vi "Data_Acquisition.vi"(0 "Upper_Limit":dbl=100.0, 5 "Lower_Bound":dbl, 11 "Error_In":errorcluster) -> (4 "Generated_Number":dbl, 15 "Error_Out":errorcluster)   [LabVIEW 2021]
doc: "This VI Generate data and transmit it to other vi through Queue and stack"
uses:
  Controls/Operation_Select_Queue.ctl
  Controls/Data.ctl
  Controls/Operation_Select_Stack.ctl
  <vilib>/numeric/Random Number (Range) DBL.vi
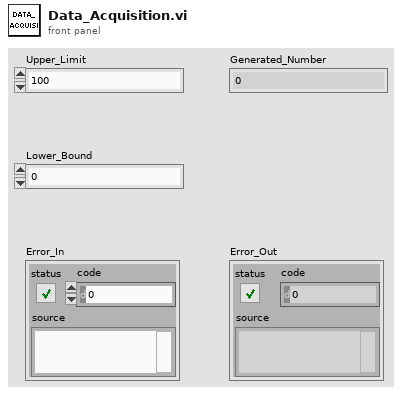
[diagram p1: front panel]
types:
  T1 = typedef "Operation_Select_Stack.ctl" = enum16{"Initialize", "Push", "Pop", "Preview"}
  T2 = typedef "Data.ctl" = cluster{"Generated_Data":dbl, "Time_Stamp":string}
  T3 = typedef "Operation_Select_Queue.ctl" = enum16{"Initialize", "Enqueue", "Dequeue", "Preview"}
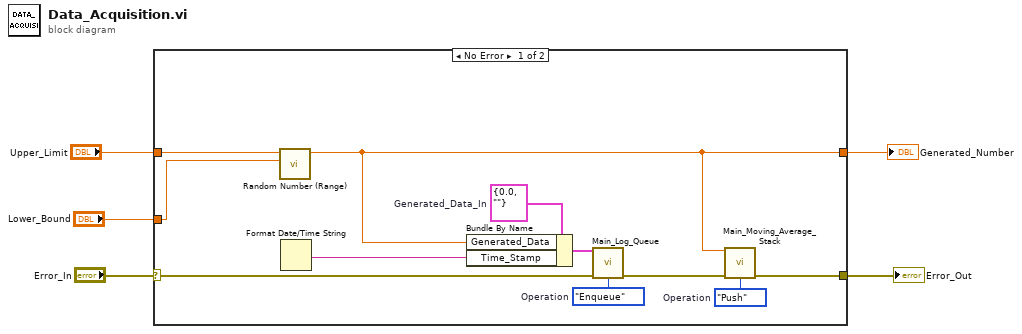
[diagram p0: block diagram]
diagram:
  n1 = case shown="No Error" "Error_In" {
    selector: "Error_In" -> [w15 w17]
    tunnel: [w14 w17] -> w4
    tunnel: [w10 _] -> w3
    tunnel: "Upper_Limit" -> [w7 _]
    tunnel: "Lower_Bound" -> [w6 _]
    frame No Error {
      w8 = Operation_Select_Stack."Push"  # Operation
      w12 = T2 {"Generated_Data"=0.0, "Time_Stamp"=""}  # Generated_Data_In
      w13 = Operation_Select_Queue."Enqueue"  # Operation
      n2 = call-poly <vilib>:"Random Number (Range).vi"("lower bound (0)"=w6, "upper bound (100)"=w7) -> ("number"=w10:dbl)  [unwired: 9 in]
      n3 = Format Date/Time String() -> (date/time string=w9:string)  [unwired: 3 in]
      n4 = Bundle By Name(cluster=w12, "Generated_Data"=w10, "Time_Stamp"=w9) -> (w11:T2)
      n5 = call "Main_Log_Queue.vi"("Generated_Data_In"=w11, "Error_In"=w15, "Operation"=w13) -> ("Error_Out"=w16:errorcluster)  [unwired: 8 in, 4 out]
      n6 = call "Main_Moving_Average_Stack.vi"("Generated_Data_In"=w10, "Error_In"=w16, "Operation"=w8) -> ("Error_Out"=w14:errorcluster)  [unwired: 8 in, 4 out]
    }
    frame Error {
    }
  }
  "Error_Out" <- w4
  "Generated_Number" <- w3
